vi "Write Device List State to File.vi"(8 "Error In":errorcluster, 10 "file path":path, 11 "Device List State":T1) -> (0 "Error Out":errorcluster, 2 "file path out":path, 3 "Device List State out":T1)   [LabVIEW 2015]
uses:
  Device List State.ctl
  Device/Device.lvclass
  Dynamic FP XControl/Name type and data.ctl
  Device/Device type.ctl
  Device/Read Controls Snapshot.vi
  Device/Read Name.vi
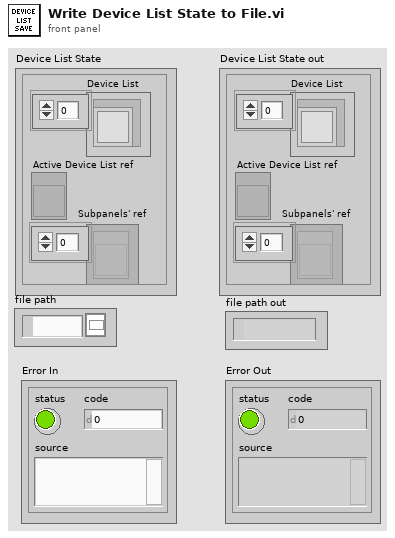
[diagram p1: front panel]
types:
  T1 = typedef "Device List State.ctl" = cluster{"Device List":refnum<class "Device.lvclass">[], "Active Device List ref":refnum<vi>, "Subpanels' ref":refnum<vi>[]}
  T2 = typedef "Name type and data.ctl" = cluster{"Front Panel Data":variant, "Device type":T3, "Name":string}
  T3 = typedef "Device type.ctl" = enum16{"NONE", "Neocera 21", "LakeShore 335", "LakeShore 340", "LkShr 340 chA&B", "LakeShore 370", "SRS 850", "SRS 830", "LR 700", "EG&G 5302", "EG&G 7260", "EG&G 7280", "AH 2500", "Keithley meter", "Keithley electrometer", "Keithley 182", "HP 5385", "HP 53181", "HP 53132", "ITC503", "IPS120", "Oxford Mercury IPS", "Oxford PS", "Test", "DC Facility Magnet", "Cryomagnetics PS", "Keithley 2400", "Keithley current source", "Cryo-Con 22C", "HP87NN", "HP4395A"}
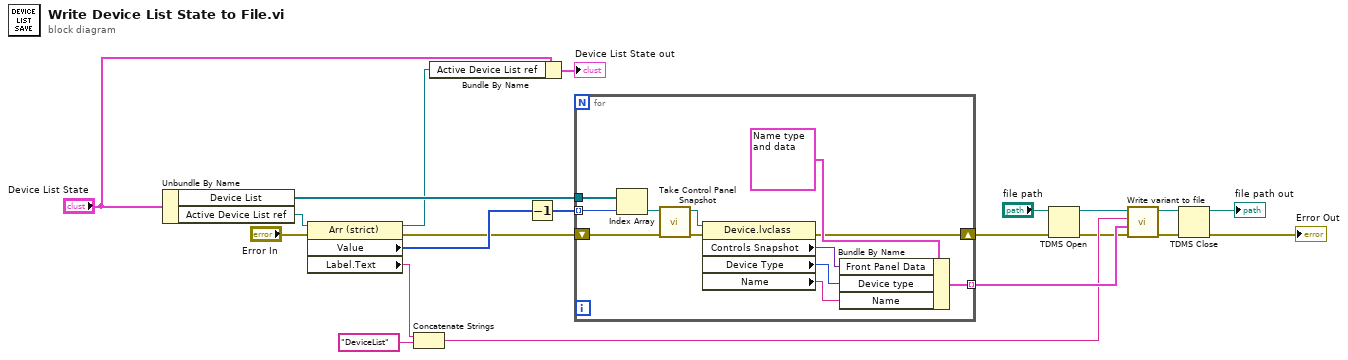
[diagram p0: block diagram]
diagram:
  n1 = Unbundle By Name("Device List State") -> ("Device List"=w15:refnum<class "Device.lvclass">[], "Active Device List ref"=w18:refnum<vi>)
  n2 = property class="Arr (strict)"(reference=w18, error in="Error In") -> (reference out=w11:refnum<vi>, error out=w12:errorcluster, "Value"=w17:u16[], "Label.Text"=w8:string)
  n3 = Concatenate Strings(w8, "DeviceList" ("string")) -> (w13:string)
  n4 = Bundle By Name(cluster="Device List State", "Active Device List ref"=w11) -> (→"Device List State out":T1)
  n5 = Decrement(x=w17) -> (x-1=w16:u16[])
  n6 = for {
    tunnel: w16 -> [w33] mode=indexing
    tunnel: w15 -> [w32]
    tunnel: [w25] -> w14 mode=indexing
    shift-right: [w22] -> w5
    shift-left: w12 -> [w24]
    n7 = Index Array(array=w32, index=w33) -> (element=w29:refnum<class "Device.lvclass">)
    n8 = call-dynamic "Take Control Panel Snapshot.vi"("error in (no error)"=w24, "Device in"=w29) -> ("error out"=w23:errorcluster, "Device out"=w30:refnum<class "Device.lvclass">)  [unwired: 7 in, 1 out]
    n9 = property class="Device.lvclass"(reference=w30, error in=w23) -> (error out=w22:errorcluster, "Controls Snapshot"=w28:variant, "Device Type"=w27:T3, "Name"=w26:string)  [unwired: 1 out]
    n10 = Bundle By Name(cluster=T2 {"Front Panel Data"=variant, "Device type"=enum."NONE", "Name"=""} ("Name type and data"), "Front Panel Data"=w28, "Device type"=w27, "Name"=w26) -> (w25:T2)
  }
  n11 = TDMS Open(8:w5, 11:"file path") -> (0:w6:errorcluster, 3:w4:refnum<k34>)  [unwired: 5 in]
  n12 = call "Write variant to file.vi"("error in (no error)"=w6, "variant"=w14, "Group name"=w13, "tdms file"=w4) -> ("error out"=w9:errorcluster, "tdms file out"=w2:refnum<k34>)  [unwired: 6 in]
  n13 = TDMS Close(8:w9, 11:w2) -> (0:→"Error Out":errorcluster, 3:→"file path out":path)
